vi "ValueChanged Event Callback.vi"(4 "User Parameter":variant, 5 "Event Data":cluster{"sender":refnum<k24>, "e":refnum<k24>}, 6 "Control Ref":refnum<k24>, 7 "Event Common Data":T1) -> ()   [LabVIEW 2024, in "MyEventGrid.lvclass"]
uses:
  MyEventGrid.lvclass
  D:/git/Sourcegrid-LabVIEW/dll/SourceGrid.dll
  dll/SourceGrid.dll
panel:
  out "variant":variant
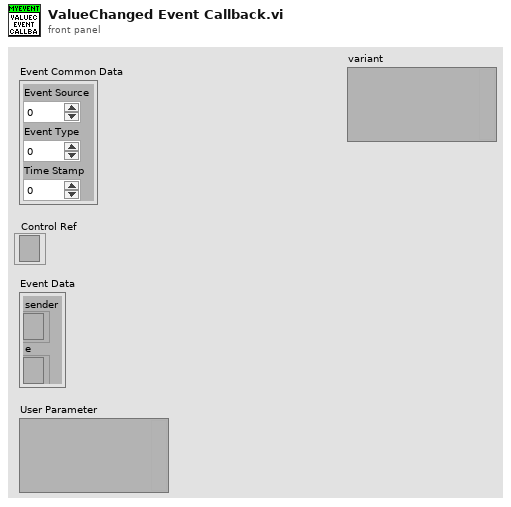
[diagram p1: front panel]
types:
  T1 = cluster{"Event Source":i32, "Event Type":u32, "Time Stamp":u32}
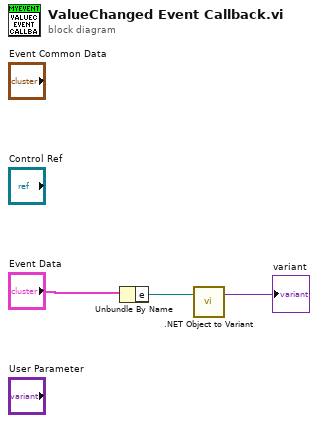
[diagram p0: block diagram]
diagram:
  n1 = Unbundle By Name("Event Data") -> ("e"=w2:refnum<k24>)
  n2 = call <vilib>:".NET Object to Variant.vi"(".NET object"=w2) -> ("variant"=→"variant":variant)  [unwired: 1 in, 1 out]
